vi "Delete Tree Items.vi"(6 "Try to delete parent as well":bool=TRUE, 7 "Num of Items to Remove":i32, 8 "Child String":string, 9 "Parent String":string, 10 "Settings In":T1[](array[typedef]) {"Data Type" items=["Tree Parent"=-1, "Numeric"=0, "String"=1, "Boolean"=2, "Enum"=3]}, 11 "Tags In":string[](array[string])) -> (2 "Settings Out":T1[](array[typedef]) {"Data Type" items=["Tree Parent"=-1, "Numeric"=0, "String"=1, "Boolean"=2, "Enum"=3]}, 3 "Tags Out":string[](array[string]))   [LabVIEW 2020, in "Sequencer with Output Values.lvlib" / "Sequencer with Output Values.lvclass"]
uses:
  Sequencer with Output Values.lvclass
  Tree Item Settings.ctl
  Data Type.ctl
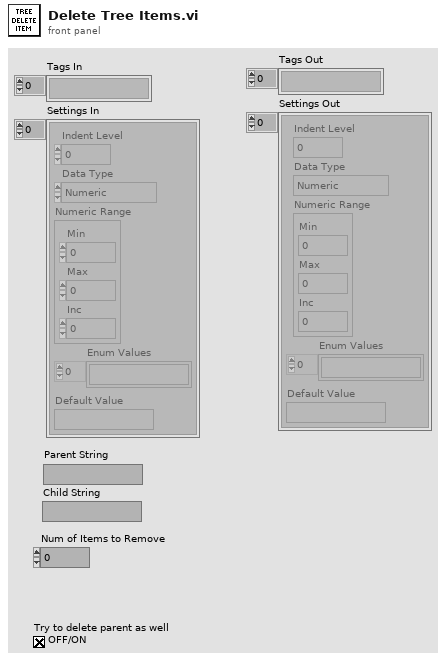
[diagram p1: front panel]
types:
  T1 = typedef "Sequencer with Output Values.lvlib/Sequencer with Output Values.lvclass/Tree Item Settings.ctl" = cluster{"Indent Level":i32, "Data Type":T2, "Numeric Range":cluster{"Min":dbl, "Max":dbl, "Inc":dbl}, "Enum Values":string[], "Default Value":string}
  T2 = typedef "Sequencer with Output Values.lvlib/Sequencer with Output Values.lvclass/Data Type.ctl" = i16
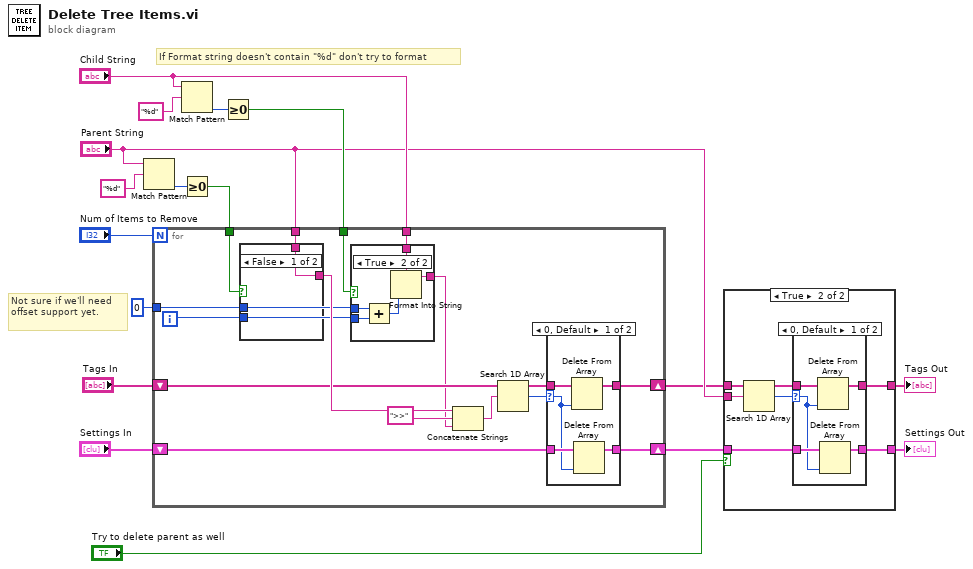
[diagram p0: block diagram]
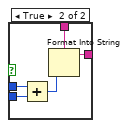
[diagram p5: hidden frame]
diagram:
  # "Not sure if we'll need offset support yet."
  # "If Format string doesn't contain \"%d\" don't try to format"
  n1 = Match Pattern(string="Parent String", regular expression="%d") -> (offset past match=w13:i32)  [unwired: 1 in, 3 out]
  n2 = Match Pattern(string="Child String", regular expression="%d") -> (offset past match=w9:i32)  [unwired: 1 in, 3 out]
  n3 = Greater Or Equal To 0?(x=w13) -> (x >= 0?=w12:bool)
  n4 = Greater Or Equal To 0?(x=w9) -> (x >= 0?=w8:bool)
  n5 = for {
    N: "Num of Items to Remove" -> [_]
    shift-right: [w27] -> w5
    shift-left: "Tags In" -> [w28]
    shift-right: [w25] -> w4
    shift-left: "Settings In" -> [w26]
    tunnel: 0 ("Start Index") -> [w19]
    tunnel: "Child String" -> [w22]
    tunnel: w12 -> [w24]
    tunnel: "Parent String" -> [w23]
    tunnel: w8 -> [w21]
    i -> [w20]
    n6 = case shown="False" w24 {
      tunnel: [w39 w44] -> w32
      tunnel: w20 -> [_ w42]
      tunnel: w19 -> [_ w41]
      tunnel: w23 -> [w39 w40]
      frame False {
      }
      frame True {
        n7 = Add(x=w41, y=w42) -> (x+y=w43:i32)
        n8 = Format Into String(format string=w40, w43) -> (resulting string=w44:string)  [unwired: 2 in, 1 out]
      }
    }
    n9 = case shown="True" w21 {
      tunnel: [w33 w38] -> w18
      tunnel: w20 -> [_ w36]
      tunnel: w19 -> [_ w35]
      tunnel: w22 -> [w33 w34]
      frame False {
      }
      frame True {
        n10 = Add(x=w35, y=w36) -> (x+y=w37:i32)
        n11 = Format Into String(format string=w34, w37) -> (resulting string=w38:string)  [unwired: 2 in, 1 out]
      }
    }
    n12 = Concatenate Strings(w32, ">>" ("string"), w18) -> (w29:string)
    n13 = Search 1D Array(1D array=w28, element=w29) -> (index of element=w30:i32)  [unwired: 1 in]
    n14 = case shown="0, Default" w30 {
      selector: w30 -> [w47 _]
      tunnel: w26 -> [w48 w50]
      tunnel: w28 -> [w49 w51]
      tunnel: [w46 w51] -> w27
      tunnel: [w45 w50] -> w25
      frame 0, Default {
        n15 = Delete From Array(array=w49, index=w47) -> (array with subset deleted=w46:string[])  [unwired: 1 in, 1 out]
        n16 = Delete From Array(array=w48, index=w47) -> (array with subset deleted=w45:T1[])  [unwired: 1 in, 1 out]
      }
      frame -1 {
      }
    }
  }
  n17 = case shown="True" "Try to delete parent as well" {
    tunnel: "Parent String" -> [_ w59]
    tunnel: w5 -> [w53 w58]
    tunnel: w4 -> [w52 w56]
    tunnel: [w53 w55] -> w3
    tunnel: [w52 w54] -> w2
    frame False {
    }
    frame True {
      n18 = Search 1D Array(1D array=w58, element=w59) -> (index of element=w57:i32)  [unwired: 1 in]
      n19 = case shown="0, Default" w57 {
        selector: w57 -> [w62 _]
        tunnel: w56 -> [w63 w65]
        tunnel: w58 -> [w64 w66]
        tunnel: [w61 w66] -> w55
        tunnel: [w60 w65] -> w54
        frame 0, Default {
          n20 = Delete From Array(array=w64, index=w62) -> (array with subset deleted=w61:string[])  [unwired: 1 in, 1 out]
          n21 = Delete From Array(array=w63, index=w62) -> (array with subset deleted=w60:T1[])  [unwired: 1 in, 1 out]
        }
        frame -1 {
        }
      }
    }
  }
  "Tags Out" <- w3
  "Settings Out" <- w2
